vi "RT AI DAQ.vi"(11 "Queue ref":T1) -> ()   [LabVIEW 2022 SP3]
uses:
  RT Controls/RT All Queue.ctl
  RT Controls/RT DAQ case.ctl
  RT Controls/RT All Loop Status.ctl
  <vilib>/DAQmx/read.llb/DAQmx Read (Analog 1D Wfm NChan NSamp).vi
  RT Create Task/RT AI Create Task.vi
  <vilib>/DAQmx/configure/timing.llb/DAQmx Timing (Sample Clock).vi
  RT Sub VI's/RT Global.vi
  <vilib>/DAQmx/miscellaneous.llb/DAQmx Fill In Error Info.vi
  <vilib>/DAQmx/configure/trigger.llb/DAQmx Start Trigger (Time).vi
panel:
  out "x-y":u32
  out "error out":errorcluster
  # "TC channel list"
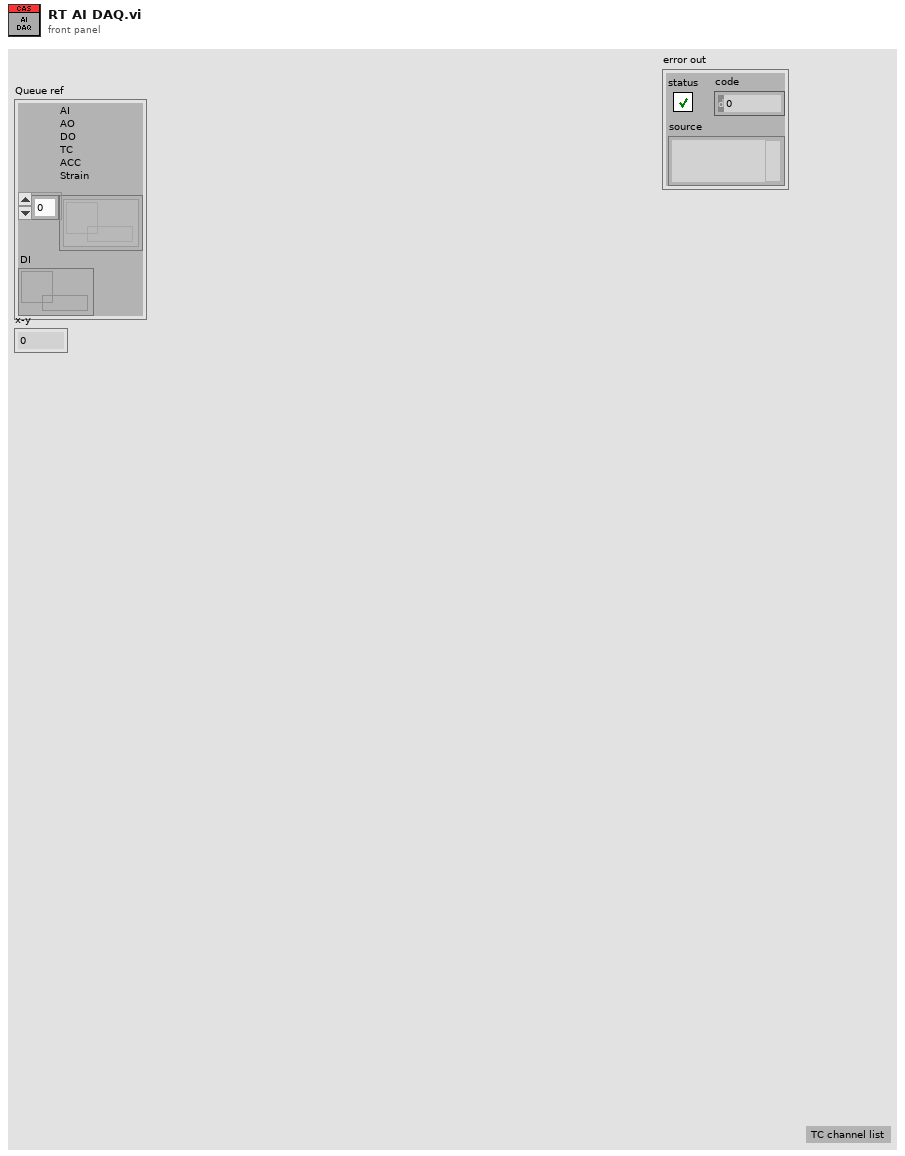
[diagram p1: front panel]
types:
  T1 = typedef "RT All Queue.ctl" = cluster{"AI\nAO\nDO\nTC\nACC\nStrain":refnum<queue>[], "DI":refnum<queue>}
  T2 = cluster{"in progress?":bool, "Start DAQ":refnum<notifier>, "task out":refnum<k21>, "AI Ref":refnum<queue>, "SPC":i32}
  T3 = typedef "RT DAQ case.ctl" = enum16{"Initailise", "Create Task", "Polevent", "Acquire", "Stop DAQ", "Error", "Exit"}
  T4 = typedef "RT All Loop Status.ctl" = enum16{"AI", "AO", "DI", "DO", "TC", "Strain", "ACC", "RT", "Log", "Seq", "Sync"}
  T5 = enum16{"Init", "Read 'All'", "Read 'n'", "Read '1'", "Write '1'", "Write 'n'", "Write 'All'"}
  T6 = typedef "RT All Notifer.ctl" = cluster{"Start DAQ":refnum<notifier>, "Sequence":refnum<notifier>}
  T7 = cluster{"Analog input":bool, "Analog Output":bool, "Digital input":bool, "Digital output":bool, "Thermocouple":bool, "Strain Gauge":bool, "Accelerometer":bool}
  T8 = typedef "RT Config.ctl" = cluster{"AO config":cluster{"Channel_Name":string, "Channel_Number":string, "Default_Value":dbl, "Units":string}[], "AI config":cluster{"Channel_Name":string, "Channel_Number":string, "Pre_Scale_min":dbl, "Pre_Scale_max":dbl, "Sensor_min":dbl, "Sensor_max":dbl, "Units":string}[], "DI config":cluster{"Channel_Name":string, "Channel_Number":string, "Default_Value":bool, "Units":bool}[], "DO config":cluster{"Channel_Name":string, "Channel_Number":string, "Default_Value":bool, "Units":bool}[], "TC config":cluster{"Channel_Name":string, "Channel_Number":string, "Pre_Scale_min":dbl, "Pre_Scale_max":dbl, "units":i32, " type":i32}[], "ACC config":cluster{"Channel_Name":string, "Channel_Number":string, "Pre_Scale_min":dbl, "Pre_Scale_max":dbl, "Terminal configuration":i32, "Sensitivity":dbl, "Sensitivity units":i32}[], "SG config":cluster{"Channel_Name":string, "Channel_Number":string, "Pre_Scale_min":dbl, "Pre_Scale_max":dbl}[], "Strain Gauge Settings":cluster{"poisson ratio":dbl, "nominal gage resistance":dbl, "gage factor":dbl}, "Bridge Settings ":cluster{"strain configuration":i32, "lead wire resistance":dbl, "initial bridge voltage":dbl, "voltage excitation source":i32, "voltage excitation value":dbl}, "Sample Rate":cluster{"AI Sample Rate":dbl, "AO Sample Rate":dbl, "DI Sample Rate":dbl, "TC Sample Rate":dbl, "DO Sample Rate":dbl, "SG Sample Rate":dbl, "ACC Sample Rate":dbl}}
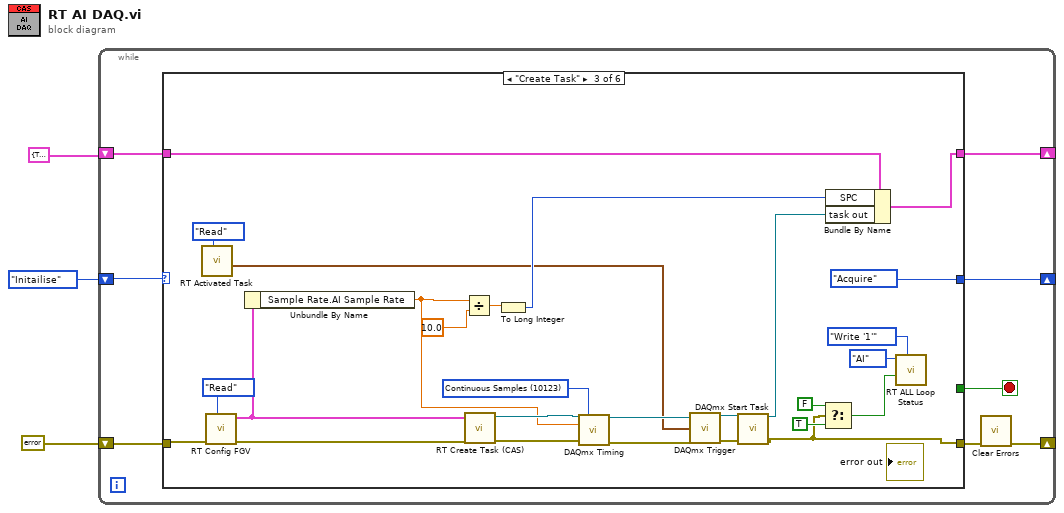
[diagram p0: block diagram]
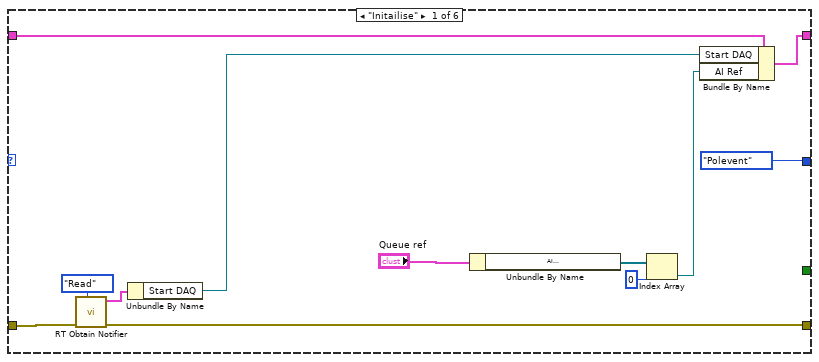
[diagram p2: hidden frame]
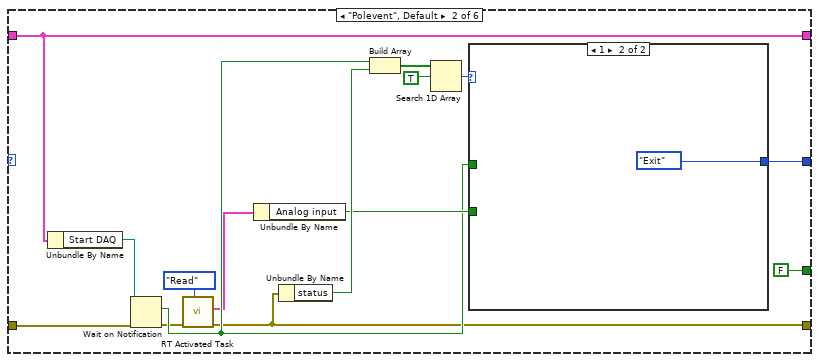
[diagram p3: hidden frame]
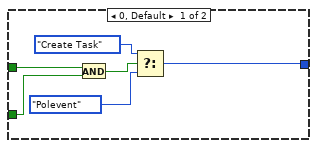
[diagram p4: hidden frame]
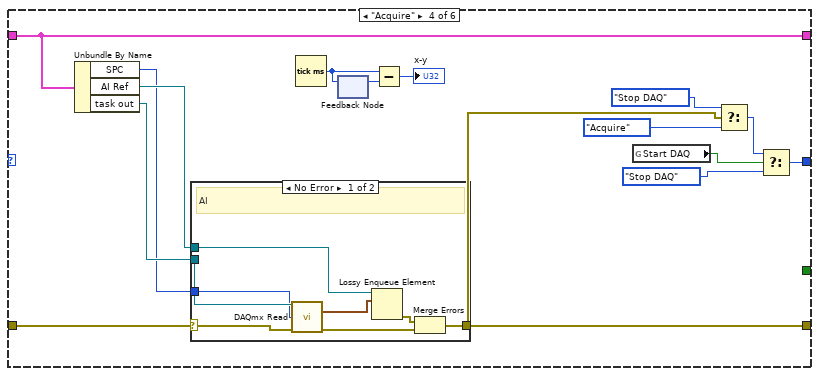
[diagram p5: hidden frame]
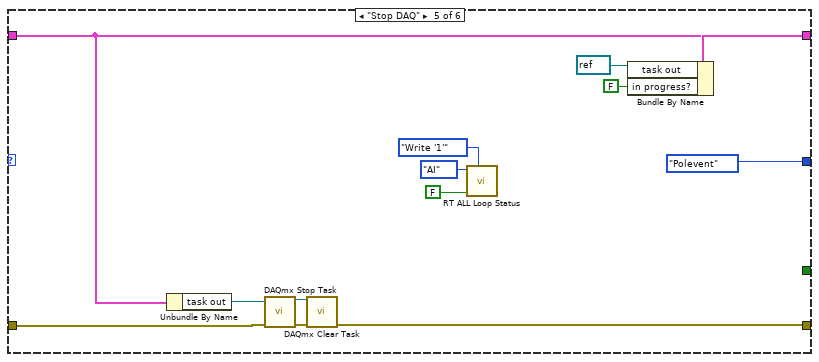
[diagram p7: hidden frame]
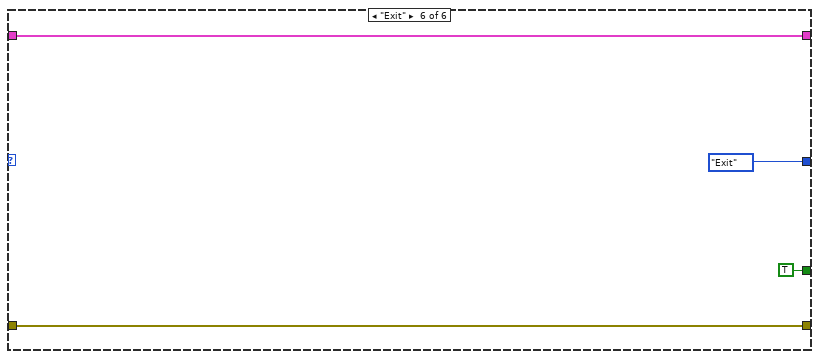
[diagram p8: hidden frame]
diagram:
  n1 = while {
    shift-right: [w4] -> _
    shift-left: errorcluster {"status"=FALSE, "code"=0, "source"=""} ("error out") -> [w10]
    shift-right: [w8] -> _
    shift-left: T2 {"in progress?"=TRUE, "Start DAQ"=refnum, "task out"="", "AI Ref"=refnum, "SPC"=0} -> [w9]
    shift-right: [w7] -> _
    shift-left: RT_DAQ_case."Initailise" -> [w6]
    stop <- w11 stop-if-true
    n2 = case shown="\"Create Task\"" w6 {
      tunnel: [_ FALSE _ _ _ TRUE] -> w11
      tunnel: w10 -> [w14 w28 w64 w81 w103 w113]
      tunnel: [w13 w24 w67 w78 w104 w113] -> w5
      tunnel: w9 -> [w23 w36 w72 w82 w108 w112]
      tunnel: [w21 w36 w71 w82 w109 w112] -> w8
      tunnel: [RT_DAQ_case."Polevent" w37 RT_DAQ_case."Acquire" w83 RT_DAQ_case."Polevent" RT_DAQ_case."Exit"] -> w7
      frame "Initailise" {
        n3 = call "RT Obtain Notifier.vi"("Case"=enum16{"Obtain", "Read"}."Read", "error in (no error)"=w14) -> ("error out"=w13:errorcluster, "All Notifier"=w12:T6)  [unwired: 8 in]
        n4 = Unbundle By Name(w12) -> ("Start DAQ"=w22:refnum<notifier>)
        n5 = Unbundle By Name("Queue ref") -> ("AI\nAO\nDO\nTC\nACC\nStrain"=w19:refnum<queue>[])
        n6 = Index Array(array=w19, index=0) -> (element=w18:refnum<queue>)
        n7 = Bundle By Name(cluster=w23, "Start DAQ"=w22, "AI Ref"=w18) -> (w21:T2)
      }
      frame "Polevent", Default {
        n8 = Unbundle By Name(w36) -> ("Start DAQ"=w35:refnum<notifier>)
        n9 = Wait on Notification(notifier=w35, error in (no error)=w28) -> (notification=w29:bool, error out=w25:errorcluster)  [unwired: 2 in, 2 out]
        n10 = call "RT Activated Task.vi"("Enum"=enum16{"Read", "Write"}."Read", "error in (no error)"=w25) -> ("error out"=w24:errorcluster, "Activate Task 2"=w27:T7)  [unwired: 7 in, 1 out]
        n11 = Unbundle By Name(w27) -> ("Analog input"=w30:bool)
        n12 = Unbundle By Name(w24) -> ("status"=w34:bool)
        n13 = Build Array(w29, w34) -> (w33:bool[])
        n14 = Search 1D Array(1D array=w33, element=TRUE) -> (index of element=w31:i32)  [unwired: 1 in]
        n15 = case shown="1" w31 {
          tunnel: [w44 RT_DAQ_case."Exit"] -> w37
          tunnel: w30 -> [w42 _]
          tunnel: w29 -> [w41 _]
          frame 0, Default {
            n16 = And(x=w41, y=w42) -> (x .and. y?=w43:bool)
            n17 = Select(t=RT_DAQ_case."Create Task", s=w43, f=RT_DAQ_case."Polevent") -> (s? t:f=w44:T3)
          }
          frame 1 {
          }
        }
      }
      frame "Create Task" {
        w70 = 10123 items=["Finite Samples"=10178, "Continuous Samples"=10123, "Hardware Timed Single Point"=12522] ("sample mode")
        n18 = call "RT Activated Task.vi"("Enum"=enum16{"Read", "Write"}."Read") -> ("Start Time"=w47:timestamp)  [unwired: 8 in, 2 out]
        n19 = call "RT Config FGV.vi"("Enum"=enum16{"Read", "Write"}."Read", "error in (no error)"=w64) -> ("error out"=w63:errorcluster, "Data out"=w56:T8)  [unwired: 8 in]
        n20 = Unbundle By Name(w56) -> ("Sample Rate.AI Sample Rate"=w55:dbl)
        n21 = Divide(x=w55, y=10.0) -> (x/y=w53:dbl)
        n22 = call-poly "RT Create Task (CAS).vi"("error in"=w63, "Config"=w56) -> ("error out"=w62:errorcluster, "AI Task"=w61:refnum<k21>)  [unwired: 7 in, 1 out]
        n23 = To Long Integer(number=w53) -> (32bit integer=w52:i32)
        n24 = call-poly <vilib>:"DAQmx Timing.vi"("task/channels in"=w61, "sample mode"=w70, "rate"=w55, "error in"=w62) -> ("task out"=w51:refnum<k21>, "error out"=w50:errorcluster)  [unwired: 10 in]
        n25 = call-poly <vilib>:"DAQmx Trigger.vi"("task/channels in"=w51, "when"=w47, "error in"=w50) -> ("task out"=w49:refnum<k21>, "error out"=w48:errorcluster)  [unwired: 11 in]
        n26 = call <vilib>:"DAQmx Start Task.vi"("task/channels in"=w49, "error in"=w48) -> ("task out"=w66:refnum<k21>, "error out"=w67:errorcluster)  [unwired: 12 in]
        n27 = Select(t=FALSE, s=w67, f=TRUE) -> (s? t:f=w58:bool)
        n28 = Bundle By Name(cluster=w72, "SPC"=w52, "task out"=w66) -> (w71:T2)
        n29 = call "RT ALL Loop Status.vi"("Option"=T5."Write '1'", "Status"=w58, "Loop"=RT_All_Loop_Status."AI") -> ()  [unwired: 6 in, 3 out]
      }
      frame "Acquire" {
        n30 = Unbundle By Name(w82) -> ("SPC"=w73:i32, "AI Ref"=w80:refnum<queue>, "task out"=w79:refnum<k21>)
        n31 = case shown="No Error" w81 {
          selector: w81 -> [w91 w96]
          tunnel: w79 -> [w90 _]
          tunnel: [w93 w96] -> w78
          tunnel: w80 -> [w92 _]
          tunnel: w73 -> [w88 _]
          frame No Error {
            # "AI"
            n32 = call-poly <vilib>:"DAQmx Read.vi"("task/channels in"=w90, "number of samples per channel"=w88, "error in"=w91) -> ("data"=w89:waveform(dbl)[], "error out"=w94:errorcluster)  [unwired: 10 in, 1 out]
            n33 = Lossy Enqueue Element(queue=w92, element=w89) -> (error out=w95:errorcluster)  [unwired: 1 in, 3 out]
            n34 = Merge Errors(w95, w94) -> (w93:errorcluster)
          }
          frame Error {
          }
        }
        n35 = Tick Count (ms)() -> (millisecond timer value=w87:u32)
        n36 = feedback-in #1(w87) -> ()
        n37 = feedback #1() -> (w86:u32)  [unwired: 1 in]
        n38 = Subtract(x=w87, y=w86) -> (x-y=→"x-y":u32)
        n39 = global read "RT Global.vi" "Start DAQ"() -> (w74:bool)
        n40 = Select(t=RT_DAQ_case."Stop DAQ", s=w78, f=RT_DAQ_case."Acquire") -> (s? t:f=w84:T3)
        n41 = Select(t=w84, s=w74, f=RT_DAQ_case."Stop DAQ") -> (s? t:f=w83:T3)
      }
      frame "Stop DAQ" {
        n42 = Unbundle By Name(w108) -> ("task out"=w102:refnum<k21>)
        n43 = call <vilib>:"DAQmx Stop Task.vi"("task/channels in"=w102, "error in"=w103) -> ("task out"=w101:refnum<k21>, "error out"=w105:errorcluster)  [unwired: 12 in]
        n44 = call <vilib>:"DAQmx Clear Task.vi"("task in"=w101, "error in"=w105) -> ("error out"=w104:errorcluster)  [unwired: 13 in]
        n45 = call "RT ALL Loop Status.vi"("Option"=T5."Write '1'", "Status"=FALSE, "Loop"=RT_All_Loop_Status."AI") -> ()  [unwired: 6 in, 3 out]
        n46 = Bundle By Name(cluster=w108, "task out"=refnum<k21> refnum, "in progress?"=FALSE) -> (w109:T2)
      }
      frame "Exit" {
      }
    }
    n47 = call <vilib>:"Clear Errors.vi"("error in (no error)"=w5) -> ("error out"=w4:errorcluster)  [unwired: 5 in, 1 out]
  }
